vi "Get_Current_Scan_client.vi"(0 "ADAM Ch Names":string[](array[string])=["EnFlo Tun:Ultrasonic:Fixed"]) -> (1 "Ch Description Array":T1[](array[typedef]) {"Duty" format="%.0b"; "D" format="%#_5g"; "C" format="%#_5g"; "B" format="%#_5g"; "A" format="%#_5g"}, 2 "String values":string[](array[string]), 3 "Numerical Values":dbl[](array[numeric]) format="%.9f")   [LabVIEW 2013]
uses:
  Sub VIs/ADAM Controls/Ch_description_ADAM.ctl
  Sub VIs/ADAM Controls/Module_type_ADAM.ctl
  Sub VIs/ADAM Controls/Function_ADAM.ctl
  Sub VIs/ADAM Controls/Channel_State.ctl
  Sub VIs/ADAM Controls/Calib_type_ADAM.ctl
  Sub VIs/ADAM Controls/Address.ctl
  Anemometry/Anemometry Sub Vis/Controls/Global_mode.ctl
  Anemometry/Anemometry Sub Vis/Globals/Preference_global.vi
panel:
  in  "server type":refnum<vi>
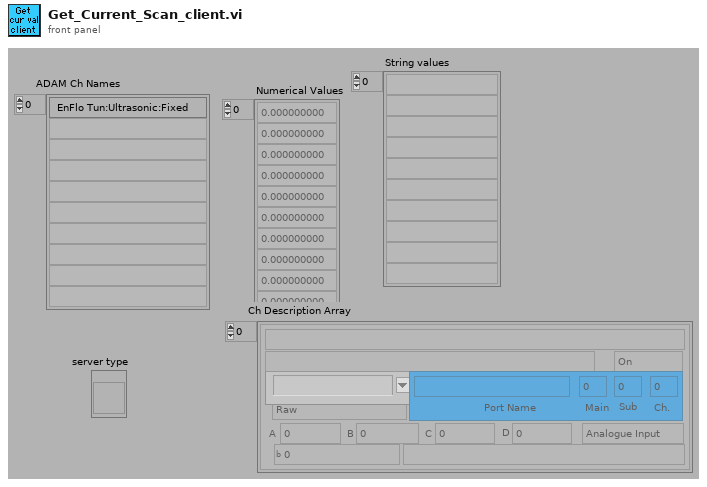
[diagram p1: front panel]
types:
  T1 = typedef "Ch_description_ADAM.ctl" = cluster{"Ch Name":string, "Type":T2, "Function":T3, "Ch State":T4, "Calibration type":T5, "A":dbl, "B":dbl, "C":dbl, "D":dbl, "Comments":string, "Address":T6, "String":string, "Duty":u16}
  T2 = typedef "Module_type_ADAM.ctl" = string
  T3 = typedef "Function_ADAM.ctl" = enum16{"Analogue Input", "Digital Input", "Event counter", "Event rate", "Analogue Output", "Digital Output", "Relay Output"}
  T4 = typedef "Channel_State.ctl" = enum16{"On", "Off", "Always On", "Always Off"}
  T5 = typedef "Calib_type_ADAM.ctl" = enum16{"Raw", "Bx + A", "Cx^2 + Bx + A", "Dx^3 + Cx^2 + Bx + A", "In Band", "Hi-Tec Q", "Hi-Tec M_dot", "Text"}
  T6 = typedef "Address.ctl" = cluster{"Main":i32, "Ch.":i32, "Sub":i32, "Port Name":string}
  T7 = typedef "Server_Comms.ctl" = enum16{"Server Link Healthy", "Do Not Link To Server"}
  T8 = typedef "Global_mode.ctl" = enum16{"Read Global", "Load Global From File", "Write Global to File"}
  T9 = typedef "Update_scan_value.ctl" = cluster{"Channel Name":string, "New Value":dbl}
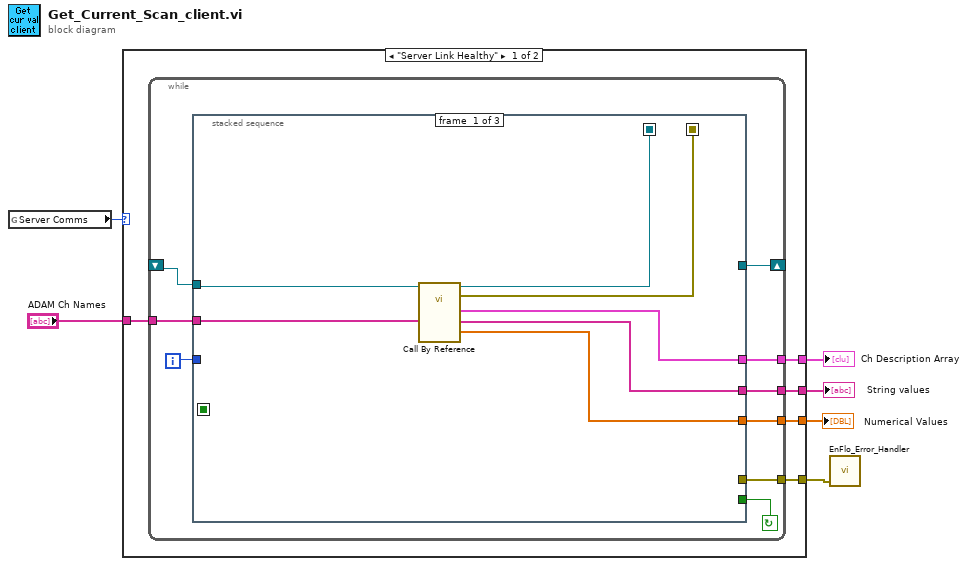
[diagram p0: block diagram]
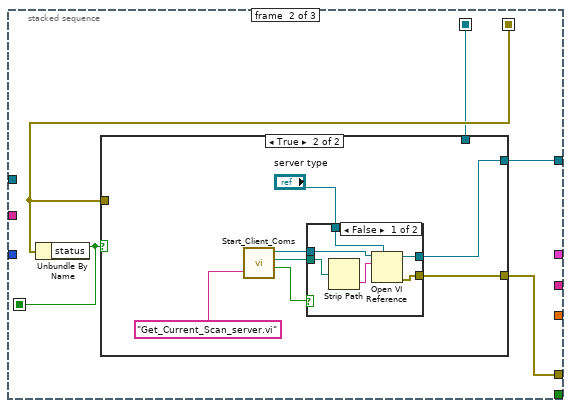
[diagram p2: hidden frame]
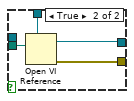
[diagram p4: hidden frame]
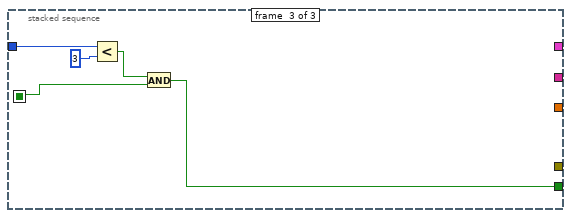
[diagram p5: hidden frame]
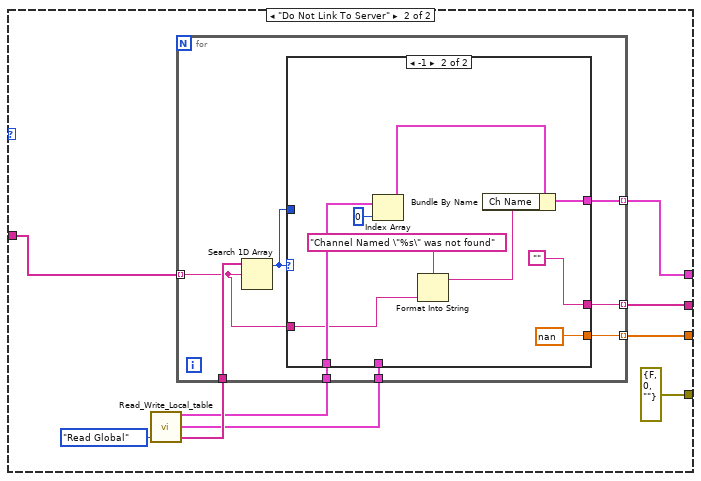
[diagram p6: hidden frame]
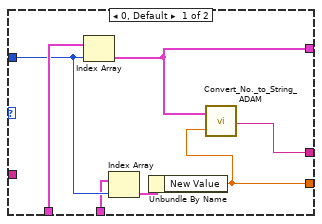
[diagram p7: hidden frame]
diagram:
  n1 = global read "Preference_global.vi" "Server Comms"() -> (w6:T7)
  n2 = case shown="\"Server Link Healthy\"" w6 {
    tunnel: [w11 errorcluster {"status"=FALSE, "code"=0, "source"=""}] -> w5
    tunnel: "ADAM Ch Names" -> [w10 w62]
    tunnel: [w7 w57] -> w1
    tunnel: [w9 w60] -> w3
    tunnel: [w8 w59] -> w2
    frame "Server Link Healthy" {
      n3 = while {
        tunnel: [w13] -> w8
        tunnel: [w14] -> w9
        tunnel: w10 -> [w15]
        tunnel: [w16] -> w11
        shift-left: _ -> [w20]
        shift-right: [w19] -> _
        tunnel: [w12] -> w7
        i -> [w18]
        stop <- w17 continue-if-true
        n4 = stacked-sequence {
          seq-local: [w25 _ _] -> [_ w28 _]
          seq-local: [w27 _ _] -> [_ w29 _]
          seq-local: [_ w31 _] -> [_ _ w53]
          tunnel: w20 -> [w26 _ _]
          tunnel: [_ w32 _] -> w19
          tunnel: w18 -> [_ _ w54]
          tunnel: [_ _ w52] -> w17
          tunnel: [_ w30 _] -> w16
          tunnel: w15 -> [w21 _ _]
          tunnel: [w23 _ _] -> w14
          tunnel: [w22 _ _] -> w13
          tunnel: [w24 _ _] -> w12
          frame #0 {
            n5 = call-by-ref "Call By Reference"(reference=w26, "Desired Channels"=w21) -> (reference out=w25:refnum<vi>, error out=w27:errorcluster, "Ch Description Array"=w24:T1[], "String values"=w23:string[], "Numerical Values"=w22:dbl[])  [unwired: 1 in]
          }
          frame #1 {
            n6 = Unbundle By Name(w29) -> ("status"=w31:bool)
            n7 = case shown="True" w31 {
              tunnel: [w33 w37] -> w32
              tunnel: [w34 w35] -> w30
              tunnel: w29 -> [w34 _]
              tunnel: w28 -> [w33 _]
              frame False {
              }
              frame True {
                n8 = call "Start_Client_Coms.vi"("VI name to run on server"="Get_Current_Scan_server.vi") -> ("LabVIEW application reference"=w39:refnum<vi>, "Checked VI name"=w40:path, "Local Call"=w38:bool)  [unwired: 1 in, 1 out]
                n9 = case shown="False" w38 {
                  tunnel: [w45 w51] -> w37
                  tunnel: "server type" -> [w44 w50]
                  tunnel: w40 -> [w43 w49]
                  tunnel: w39 -> [w42 _]
                  tunnel: [w46 w48] -> w35
                  frame False {
                    n10 = Strip Path(path=w43) -> (name=w47:string)  [unwired: 1 out]
                    n11 = Open VI Reference(type specifier VI Refnum (for type only)=w44, application reference (local)=w42, vi path=w47) -> (vi reference=w45:refnum<vi>, error out=w46:errorcluster)  [unwired: 1 in, 2 out]
                  }
                  frame True {
                    n12 = Open VI Reference(type specifier VI Refnum (for type only)=w50, vi path=w49) -> (vi reference=w51:refnum<vi>, error out=w48:errorcluster)  [unwired: 1 in, 3 out]
                  }
                }
              }
            }
          }
          frame #2 {
            n13 = Less?(x=w54, y=3) -> (x < y?=w56:bool)
            n14 = And(x=w56, y=w53) -> (x .and. y?=w52:bool)
          }
        }
      }
    }
    frame "Do Not Link To Server" {
      n15 = call "Read_Write_Local_table.vi"("Mode"=Global_mode."Read Global") -> ("Ch Names"=w63:string[], "Ch Values Out"=w58:T9[], "Channels Descriptions Out"=w61:T1[])  [unwired: 2 in]
      n16 = for {
        tunnel: w63 -> [w73]
        tunnel: w62 -> [w66] mode=indexing
        tunnel: w61 -> [w71]
        tunnel: [w70] -> w57 mode=indexing
        tunnel: [w69] -> w60 mode=indexing
        tunnel: [w68] -> w59 mode=indexing
        tunnel: w58 -> [w67]
        n17 = Search 1D Array(1D array=w73, element=w66) -> (index of element=w72:i32)  [unwired: 1 out]
        n18 = case shown="-1" w72 {
          tunnel: w72 -> [w79 _]
          tunnel: w71 -> [w80 w88]
          tunnel: [w76 w86] -> w70
          tunnel: [w74 ""] -> w69
          tunnel: [w75 nan] -> w68
          tunnel: w67 -> [w78 _]
          tunnel: w66 -> [_ w83]
          frame 0, Default {
            n19 = Index Array(array=w80, index=w79) -> (element=w76:T1)
            n20 = Index Array(array=w78, index=w79) -> (element=w77:T9)
            n21 = Unbundle By Name(w77) -> ("New Value"=w75:dbl)
            n22 = call "Convert_No._to_String_ADAM.vi"("Input number"=w75, "Ch Description"=w76) -> ("Output sting"=w74:string)
          }
          frame -1 {
            n23 = Index Array(array=w88, index=0 ("Index")) -> (element=w87:T1)
            n24 = Format Into String(format string="Channel Named \"%s\" was not found" ("Format String"), w83) -> (resulting string=w81:string)  [unwired: 2 in, 1 out]
            n25 = Bundle By Name(cluster=w87, "Ch Name"=w81) -> (w86:T1)
          }
        }
      }
    }
  }
  "Ch Description Array" <- w1
  "String values" <- w3
  "Numerical Values" <- w2
  n26 = call "EnFlo_Error_Handler.vi"("error in (no error)"=w5) -> ()  [unwired: 2 in, 3 out]
